vi "CH_LM App SetLabelUnit.vi"(0 "Unit References":T1, 1 "Mode":enum32{"Energy", "Power", "Power/dB"}(radio)=enum."Power") -> ()   [LabVIEW 2012, in "CH_LM App.lvlib"]
doc: "This VI is used to set the correct unit in the indicator labels/captions."
uses:
  CH_LM App.lvlib
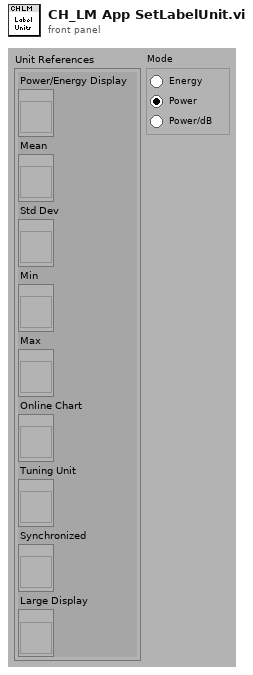
[diagram p1: front panel]
types:
  T1 = cluster{"Power/Energy Display":refnum<vi>, "Mean":refnum<vi>, "Std Dev":refnum<vi>, "Min":refnum<vi>, "Max":refnum<vi>, "Online Chart":refnum<vi>, "Tuning Unit":refnum<vi>, "Synchronized":refnum<vi>, "Large Display":refnum<vi>}
  T2 = cluster{"[0]":dbl, "[1]":dbl, "[2]":dbl, "[3]":dbl, "[4]":dbl, "[5]":dbl, "[6]":dbl, "[7]":dbl, "[8]":dbl}[]
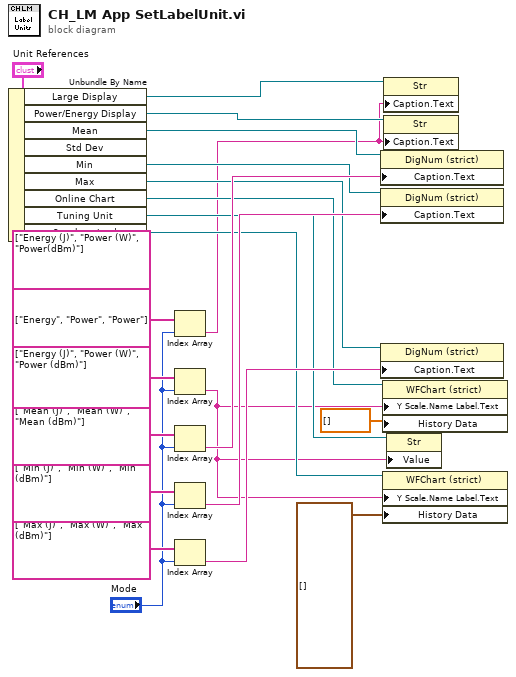
[diagram p0: block diagram]
diagram:
  (unwired) string[] ["Energy (J)", "Power (W)", "Power(dBm)"]
  n1 = Unbundle By Name("Unit References") -> ("Large Display"=w1:refnum<vi>, "Power/Energy Display"=w17:refnum<vi>, "Mean"=w16:refnum<vi>, "Min"=w14:refnum<vi>, "Max"=w12:refnum<vi>, "Online Chart"=w9:refnum<vi>, "Tuning Unit"=w8:refnum<vi>, "Synchronized"=w7:refnum<vi>)  [unwired: 1 out]
  n2 = Index Array(array=string[] ["Energy", "Power", "Power"], index="Mode") -> (element=w2:string)
  n3 = Index Array(array=string[] ["Energy (J)", "Power (W)", "Power (dBm)"], index="Mode") -> (element=w5:string)
  n4 = Index Array(array=string[] ["Mean (J)", "Mean (W)", "Mean (dBm)"], index="Mode") -> (element=w15:string)
  n5 = Index Array(array=string[] ["Min (J)", "Min (W)", "Min (dBm)"], index="Mode") -> (element=w13:string)
  n6 = Index Array(array=string[] ["Max (J)", "Max (W)", "Max (dBm)"], index="Mode") -> (element=w11:string)
  n7 = property class="DigNum (strict)"(reference=w16, "Caption.Text"=w15) -> ()  [unwired: 1 in, 2 out]
  n8 = property class="DigNum (strict)"(reference=w14, "Caption.Text"=w13) -> ()  [unwired: 1 in, 2 out]
  n9 = property class="DigNum (strict)"(reference=w12, "Caption.Text"=w11) -> ()  [unwired: 1 in, 2 out]
  n10 = property class="WFChart (strict)"(reference=w9, "Y Scale.Name Label.Text"=w5, "History Data"=dbl[] []) -> ()  [unwired: 1 in, 2 out]
  n11 = property class="WFChart (strict)"(reference=w7, "Y Scale.Name Label.Text"=w5, "History Data"=T2 []) -> ()  [unwired: 1 in, 2 out]
  n12 = property class="Str"(reference=w1, "Caption.Text"=w2) -> ()  [unwired: 1 in, 2 out]
  n13 = property class="Str"(reference=w17, "Caption.Text"=w2) -> ()  [unwired: 1 in, 2 out]
  n14 = property class="Str"(reference=w8, "Value"=w5) -> ()  [unwired: 1 in, 2 out]
